vi "Three way slider - Copy.vi"() -> ()   [LabVIEW 2012]
panel:
  in  "Slide":u8(slide) max=2 scale=0.0..2.0
  in  "stop":bool
  out "HOLD":bool
  out "OFF":bool
  out "RUN":bool
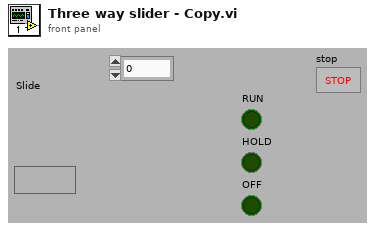
[diagram p1: front panel]
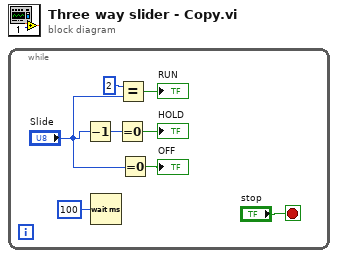
[diagram p0: block diagram]
diagram:
  n1 = while {
    stop <- "stop" stop-if-true
    n2 = Decrement(x="Slide") -> (x-1=w5:u8)
    n3 = Wait (ms)(milliseconds to wait=u32 100) -> ()  [unwired: 1 out]
    n4 = Equal To 0?(x=w5) -> (x = 0?=→"HOLD":bool)
    n5 = Equal?(x=u32 2, y="Slide") -> (x = y?=→"RUN":bool)
    n6 = Equal To 0?(x="Slide") -> (x = 0?=→"OFF":bool)
  }
